vi "Instrument Manager_Init.vi"(8 "Error In":errorcluster, 11 "reference in":refnum<class "Instrument Manager.lvclass"> caption="This control should only be used when\na sub class is inheriting this class") -> (0 "Error Out":errorcluster, 3 "reference out":refnum<class "Instrument Manager.lvclass"> caption="This indicator should only be used when\na sub class is inheriting this class")   [LabVIEW 2019, in "Instrument Manager.lvclass"]
uses:
  Instrument Manager.lvclass
  Instrument Manager.lvclass/Instrument Manager.ctl
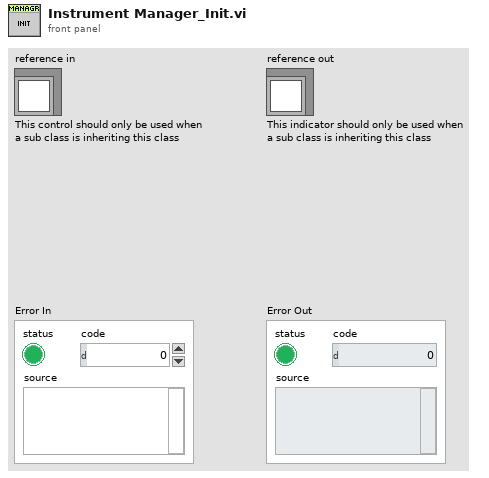
[diagram p1: front panel]
types:
  T1 = typedef "Instrument Manager.lvclass/ObjectAttributes.ctl" = cluster{"ICreate Action Point":refnum<class "ICreate Action Point.lvclass">, "IInstruments":map{string, refnum<class "IInstrument.lvclass">}, "IVirtual Instruments":map{string, refnum<class "IVirtual Instrument.lvclass">}, "Instrument Configurations":map{string, refnum<class "Config from JSON.lvclass">}, "Virtual Instrument Configurations":map{string, refnum<class "Config from JSON.lvclass">}, "Action Point Configurations":map{string, refnum<class "Config from JSON.lvclass">}, "Action Points":map{string, refnum<class "Action Point.lvclass">}}
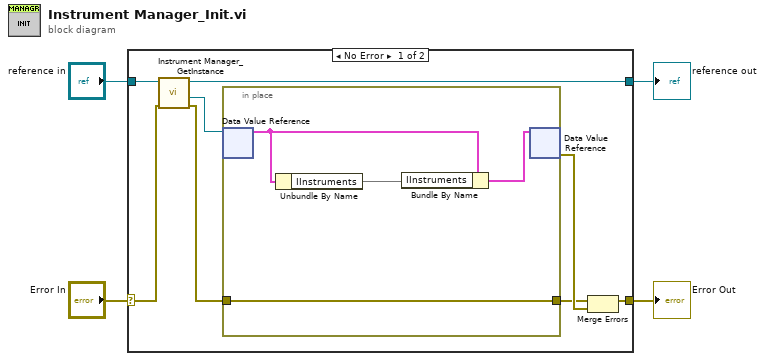
[diagram p0: block diagram]
diagram:
  n1 = case shown="No Error" "Error In" {
    selector: "Error In" -> [w10 w18]
    tunnel: [w11 w18] -> w3
    tunnel: "reference in" -> [w9 w17]
    tunnel: [w7 w17] -> w1
    frame No Error {
      n2 = call "Instrument Manager_GetInstance.vi"("Error In"=w10, "reference in"=w9) -> ("Error Out"=w6:errorcluster, "DVRRefOut"=w8:refnum<data-value>, "reference out"=w7:refnum<class "Instrument Manager.lvclass">)  [unwired: 5 in, 2 out]
      n3 = in-place {
        in-place-border: w6 -> [w13]
        in-place-border: [w13] -> w5
        n4 = in-place-dvr #1(w8) -> (w16:T1)  [unwired: 1 out]
        n5 = Unbundle By Name(w16) -> ("IInstruments"=w14:map{string, refnum<class "IInstrument.lvclass">})
        n6 = Bundle By Name(cluster=w16, "IInstruments"=w14) -> (w15:T1)
        n7 = in-place-dvr #1(w15) -> (w12:errorcluster)  [unwired: 1 out]
      }
      n8 = Merge Errors(w5, w12) -> (w11:errorcluster)
    }
    frame Error {
    }
  }
  "Error Out" <- w3
  "reference out" <- w1
